vi "CRIS requestor.vi"() -> ()   [LabVIEW 2013]
panel:
  in  "Clear Request":bool
  out "Loop Counter":i32
  out "waveReadback":dbl
  in  "Send Request":bool
  in  "WL request":dbl=10000.0 format="%#_13g"
  in  "stop":bool
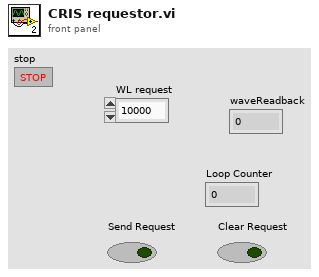
[diagram p1: front panel]
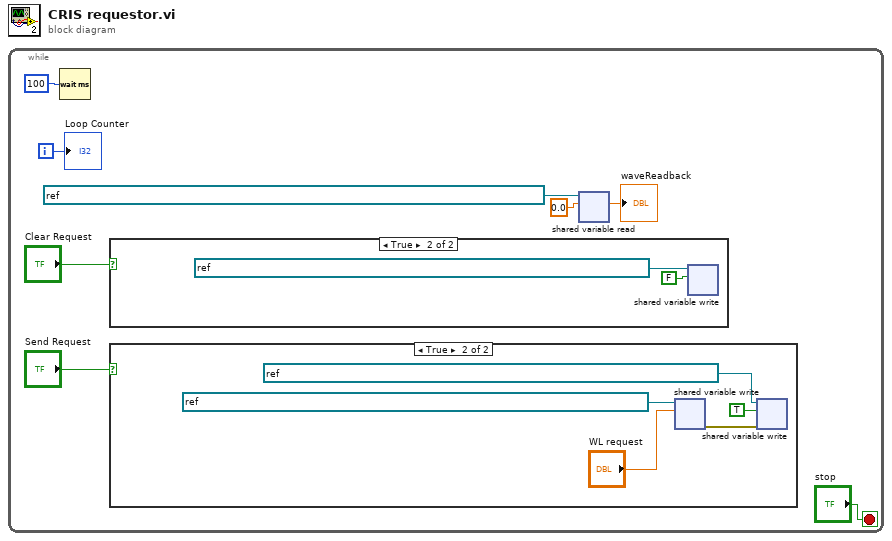
[diagram p0: block diagram]
diagram:
  n1 = while {
    i -> [w5]
    stop <- "stop" stop-if-true
    n2 = Wait (ms)(milliseconds to wait=u32 100) -> ()  [unwired: 1 out]
    n3 = case shown="True" "Clear Request" {
      frame False {
      }
      frame True {
        n4 = shared-variable-write(refnum<k21> "ni.var.psp://cwe-513-vmw172/Narrow Band TiSa Scanner Shared Variables/isNew" ("shared variable refnum in"), FALSE) -> ()  [unwired: 1 in, 2 out]
      }
    }
    n5 = case shown="True" "Send Request" {
      frame False {
      }
      frame True {
        n6 = shared-variable-write(refnum<k21> "ni.var.psp://cwe-513-vmw172/Narrow Band TiSa Scanner Shared Variables/waveSet" ("shared variable refnum in"), "WL request") -> (w14:errorcluster)  [unwired: 1 in, 1 out]
        n7 = shared-variable-write(refnum<k21> "ni.var.psp://cwe-513-vmw172/Narrow Band TiSa Scanner Shared Variables/isNew" ("shared variable refnum in"), w14, TRUE) -> ()  [unwired: 2 out]
      }
    }
    n8 = shared-variable-read(refnum<k21> "ni.var.psp://cwe-513-vmw172/Narrow Band TiSa Scanner Shared Variables/waveReadback" ("shared variable refnum in"), 0.0) -> (→"waveReadback":dbl)  [unwired: 1 in, 3 out]
    "Loop Counter" <- w5
  }
